vi "To Standard Name.vi"(8 "error in (no error)":errorcluster, 9 "zero index bit":bool=TRUE, 10 "zero index element":bool=TRUE, 11 "Channel":T1={"Name"="", "Modbus Type"=enum."Input Register", "Veristand Type"=enum."Input", "Mapping"={"DataType"=enum."Double", "Starting Address"=0, "Sub-Index (Bool)"=0, "VS Reference"=0}}) -> (0 "error out":errorcluster, 2 "standard name":string)   [LabVIEW 2020]
uses:
  Shared/Controls/Data Model/Channel.ctl
  Modbus Type.ctl
  <vilib>/NI VeriStand/Custom Device API/Custom Device Channel Type.ctl
  Shared/Controls/Data Model/Mapping.ctl
  Shared/Controls/Data Model/DataType.ctl
  <vilib>/NI VeriStand/Custom Device API/Custom Device Item Ref.ctl
  Shared/Modbus Master Shared.lvlib
  <vilib>/NI VeriStand/Custom Device API/Custom Device API.lvlib
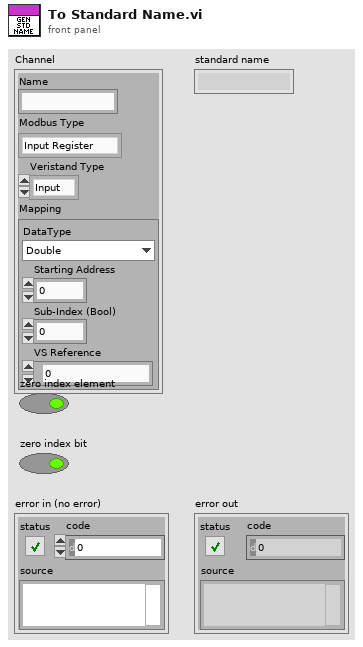
[diagram p1: front panel]
types:
  T1 = typedef "Modbus Master Shared.lvlib/Channel.ctl" = cluster{"Name":string, "Modbus Type":T2, "Veristand Type":T3, "Mapping":T4}
  T2 = typedef "Modbus Master Shared.lvlib/Modbus Type.ctl" = enum16{"Coil", "Discrete Input", "Holding Register", "Input Register"}
  T3 = typedef "Custom Device API.lvlib/Custom Device Channel Type.ctl" = enum16{"Input", "Output"}
  T4 = typedef "Modbus Master Shared.lvlib/Mapping.ctl" = cluster{"DataType":T5, "Starting Address":u16, "Sub-Index (Bool)":u16, "VS Reference":T6}
  T5 = typedef "Modbus Master Shared.lvlib/DataType.ctl" = enum16{"Double", "Single", "I64", "I32", "I16", "I8", "U64", "U32", "U16", "U8", "Boolean"}
  T6 = typedef "Custom Device API.lvlib/Custom Device Item Ref.ctl" = u64
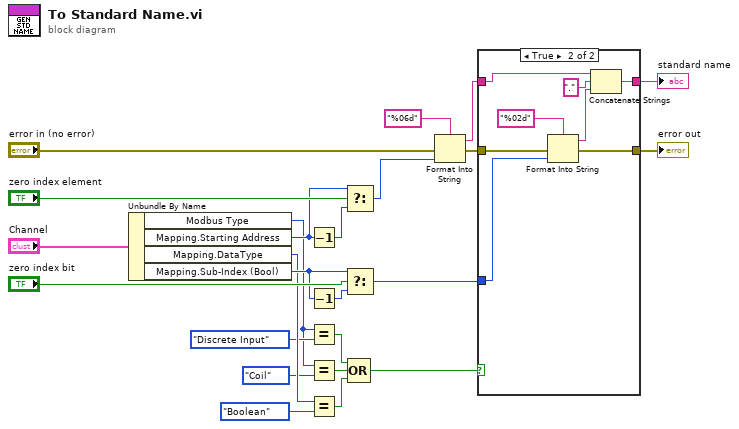
[diagram p0: block diagram]
diagram:
  n1 = Unbundle By Name("Channel") -> ("Modbus Type"=w13:T2, "Mapping.Starting Address"=w18:u16, "Mapping.DataType"=w17:T5, "Mapping.Sub-Index (Bool)"=w21:u16)
  n2 = Decrement(x=w18) -> (x-1=w20:u16)
  n3 = Decrement(x=w21) -> (x-1=w22:u16)
  n4 = Equal?(x=w13, y=Modbus_Type."Discrete Input" ("Type")) -> (x = y?=w12:bool)
  n5 = Equal?(x=w13, y=Modbus_Type."Coil" ("Type")) -> (x = y?=w11:bool)
  n6 = Equal?(x=w17, y=DataType."Boolean" ("Mapping.DataType")) -> (x = y?=w10:bool)
  n7 = Select(t=w18, s="zero index element", f=w20) -> (s? t:f=w7:u16)
  n8 = Select(t=w21, s="zero index bit", f=w22) -> (s? t:f=w5:u16)
  n9 = Compound Arithmetic op=OR(w12, w11, w10) -> (w9:bool)
  n10 = Format Into String(format string="%06d" ("initial string"), error in="error in (no error)", w7) -> (resulting string=w6:string, error out=w1:errorcluster)  [unwired: 1 in]
  n11 = case shown="True" w9 {
    tunnel: w6 -> [w26 w32]
    tunnel: w5 -> [_ w34]
    tunnel: [w26 w29] -> w4
    tunnel: [w25 w27] -> w2
    tunnel: w1 -> [w25 w28]
    frame False {
    }
    frame True {
      n12 = Format Into String(format string="%02d" ("initial string"), error in=w28, w34) -> (resulting string=w30:string, error out=w27:errorcluster)  [unwired: 1 in]
      n13 = Concatenate Strings(w32, "." ("string"), w30) -> (w29:string)
    }
  }
  "standard name" <- w4
  "error out" <- w2
